vi "开关变量转字符串.vi"(3 "板子选择":bool, 4 "bit0":bool, 5 "bit2":bool, 6 "bit1":bool, 7 "复位芯片bit3":bool, 8 "校准bit4":bool, 9 "重置输出信号bit5":bool, 10 "调试模式bit6":bool, 11 "开启控制bit7":bool) -> (1 "输出字符串":string)   [LabVIEW 2017]
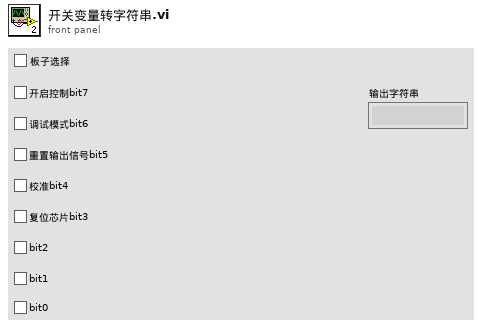
[diagram p1: front panel]
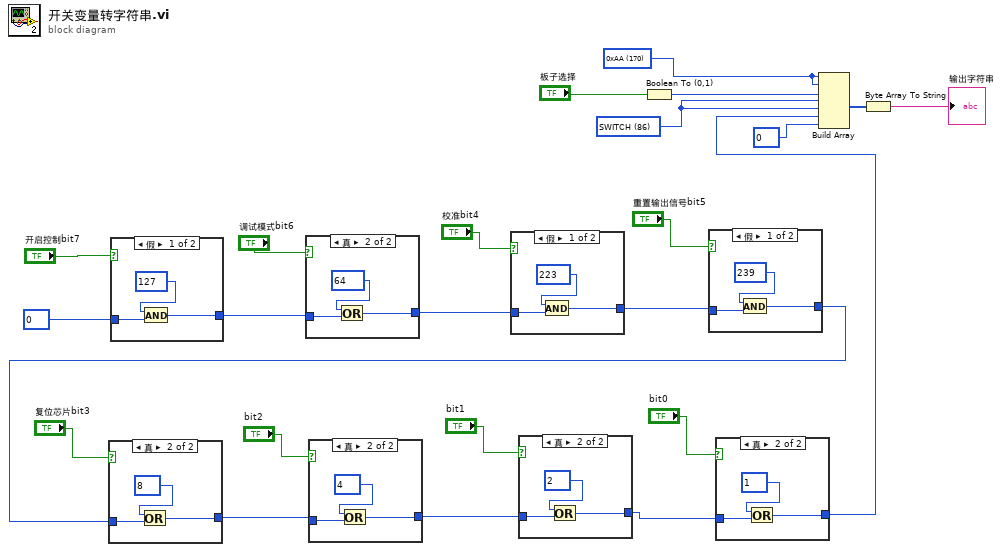
[diagram p0: block diagram]
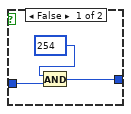
[diagram p2: hidden frame]
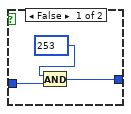
[diagram p3: hidden frame]
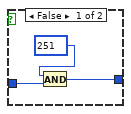
[diagram p4: hidden frame]
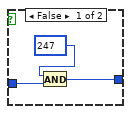
[diagram p5: hidden frame]
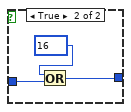
[diagram p6: hidden frame]
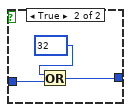
[diagram p7: hidden frame]
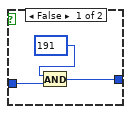
[diagram p8: hidden frame]
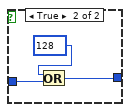
[diagram p9: hidden frame]
diagram:
  w22 = u16 170 items=["0xAA"=170, "CH0"=0, "CH1"=1, "CH01"=2, "CARLIB"=85, "SWITCH"=86, "CONTROL"=87]
  w21 = u16 86 items=["0xAA"=170, "CH0"=0, "CH1"=1, "CH01"=2, "CARLIB"=85, "SWITCH"=86, "CONTROL"=87]
  n1 = case shown="假" "开启控制bit7" {
    tunnel: 0 -> [w26 w30]
    tunnel: [w25 w28] -> w19
    frame False {
      n2 = And(x=127, y=w26) -> (x .and. y?=w25:i32)
    }
    frame True {
      n3 = Or(x=128, y=w30) -> (x .or. y?=w28:i32)
    }
  }
  n4 = case shown="真" "调试模式bit6" {
    tunnel: w19 -> [w32 w36]
    tunnel: [w31 w34] -> w12
    frame False {
      n5 = And(x=191, y=w32) -> (x .and. y?=w31:i32)
    }
    frame True {
      n6 = Or(x=64, y=w36) -> (x .or. y?=w34:i32)
    }
  }
  n7 = case shown="假" "校准bit4" {
    tunnel: w12 -> [w38 w42]
    tunnel: [w37 w40] -> w10
    frame False {
      n8 = And(x=223, y=w38) -> (x .and. y?=w37:i32)
    }
    frame True {
      n9 = Or(x=32, y=w42) -> (x .or. y?=w40:i32)
    }
  }
  n10 = Boolean To (0,1)(Boolean="板子选择") -> (0, 1=w23:i16)
  n11 = case shown="假" "重置输出信号bit5" {
    tunnel: w10 -> [w44 w48]
    tunnel: [w43 w46] -> w9
    frame False {
      n12 = And(x=239, y=w44) -> (x .and. y?=w43:i32)
    }
    frame True {
      n13 = Or(x=16, y=w48) -> (x .or. y?=w46:i32)
    }
  }
  n14 = case shown="真" "复位芯片bit3" {
    tunnel: w9 -> [w50 w54]
    tunnel: [w49 w52] -> w6
    frame False {
      n15 = And(x=247, y=w50) -> (x .and. y?=w49:i32)
    }
    frame True {
      n16 = Or(x=8, y=w54) -> (x .or. y?=w52:i32)
    }
  }
  n17 = case shown="真" "bit2" {
    tunnel: w6 -> [w56 w60]
    tunnel: [w55 w58] -> w4
    frame False {
      n18 = And(x=251, y=w56) -> (x .and. y?=w55:i32)
    }
    frame True {
      n19 = Or(x=4, y=w60) -> (x .or. y?=w58:i32)
    }
  }
  n20 = case shown="真" "bit1" {
    tunnel: w4 -> [w62 w66]
    tunnel: [w61 w64] -> w2
    frame False {
      n21 = And(x=253, y=w62) -> (x .and. y?=w61:i32)
    }
    frame True {
      n22 = Or(x=2, y=w66) -> (x .or. y?=w64:i32)
    }
  }
  n23 = case shown="真" "bit0" {
    tunnel: w2 -> [w68 w72]
    tunnel: [w67 w70] -> w1
    frame False {
      n24 = And(x=254, y=w68) -> (x .and. y?=w67:i32)
    }
    frame True {
      n25 = Or(x=1, y=w72) -> (x .or. y?=w70:i32)
    }
  }
  n26 = Build Array(w22, w22, w23, w21, w21, w1, 0) -> (w24:i32[])
  n27 = Byte Array To String(unsigned byte array=w24) -> (string=→"输出字符串":string)
